vi "AngleFind.vi"(8 "Speed Sent (ft)":dbl, 9 "Distance off Ground (ft)":dbl, 10 "Distance to Target (Ground Distance) (ft)":dbl, 11 "Height of Target (ft)":dbl) -> (3 "Angle (Degrees?)":dbl)   [LabVIEW 2020]
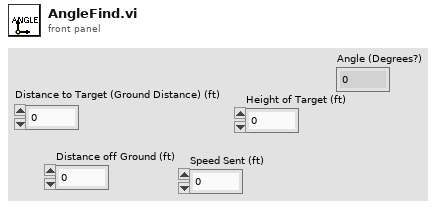
[diagram p1: front panel]
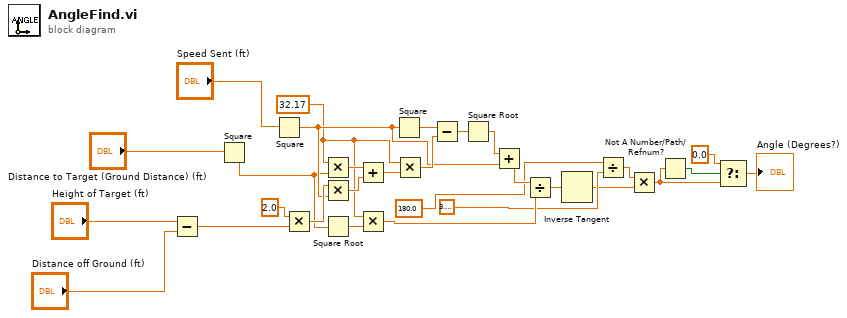
[diagram p0: block diagram]
diagram:
  w13 = 32.17
  n1 = Subtract(x="Height of Target (ft)", y="Distance off Ground (ft)") -> (x-y=w21:dbl)
  n2 = Square(x="Distance to Target (Ground Distance) (ft)") -> (x^2=w5:dbl)
  n3 = Square(x="Speed Sent (ft)") -> (x^2=w15:dbl)
  n4 = Multiply(x=2.0, y=w21) -> (x*y=w20:dbl)
  n5 = Multiply(x=w13, y=w5) -> (x*y=w23:dbl)
  n6 = Multiply(x=w20, y=w15) -> (x*y=w19:dbl)
  n7 = Square Root(x=w5) -> (sqrt(x)=w12:dbl)
  n8 = Add(x=w23, y=w19) -> (x+y=w18:dbl)
  n9 = Multiply(x=w13, y=w12) -> (x*y=w11:dbl)
  n10 = Square(x=w15) -> (x^2=w25:dbl)
  n11 = Multiply(x=w13, y=w18) -> (x*y=w26:dbl)
  n12 = Subtract(x=w25, y=w26) -> (x-y=w17:dbl)
  n13 = Square Root(x=w17) -> (sqrt(x)=w16:dbl)
  n14 = Add(x=w16, y=w15) -> (x+y=w14:dbl)
  n15 = Divide(x=w14, y=w11) -> (x/y=w10:dbl)
  n16 = Inverse Tangent(1:w10) -> (0:w6:dbl)
  n17 = Divide(x=180.0, y=3.141592653589793) -> (x/y=w7:dbl)
  n18 = Multiply(x=w7, y=w6) -> (x*y=w1:dbl)
  n19 = Not A Number/Path/Refnum?(number/path/refnum=w1) -> (NaN/Path/Refnum?=w2:bool)
  n20 = Select(t=0.0, s=w2, f=w1) -> (s? t:f=→"Angle (Degrees?)":dbl)
